vi "execution class name.vi"(8 "error in":errorcluster, 11 "Tagbus PID Module configuration in":refnum<class "PID Module configuration.lvclass">) -> (0 "error out":errorcluster, 2 "class name":string, 3 "Tagbus PID Module configuration out":refnum<class "PID Module configuration.lvclass">)   [LabVIEW 2013, in "PID Module configuration.lvclass"]
doc: "Provides an interface for determining the module runtime class associated with this module configuration. This class name can then be used to dynamically load or locate the runtime class for initialization purposes."
uses:
  PID Module configuration.lvclass
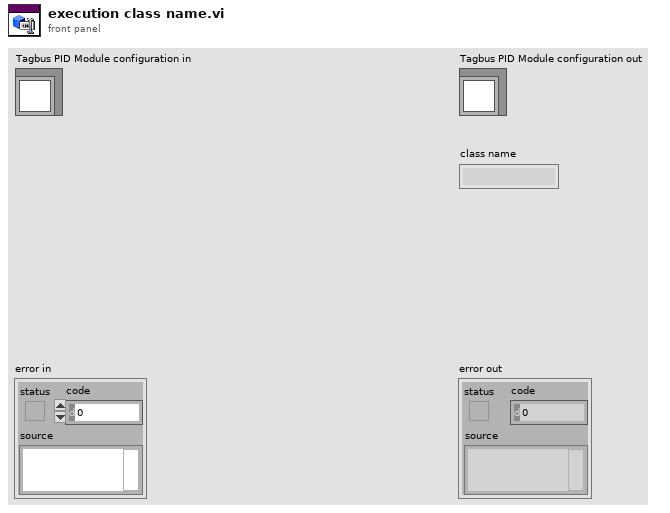
[diagram p1: front panel]
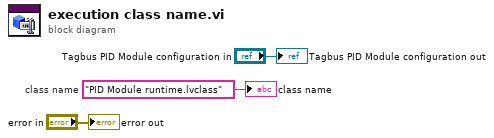
[diagram p0: block diagram]
diagram:
  w1 = "PID Module runtime.lvclass"  # class name
  "error out" <- "error in"
  "Tagbus PID Module configuration out" <- "Tagbus PID Module configuration in"
  "class name" <- w1
